vi "Experimentos de eletricidade.vi"() -> ()   [LabVIEW 2014]
panel:
  in  "Opções de aula":u16(ring) items=["Divisor de tensão.vi"]
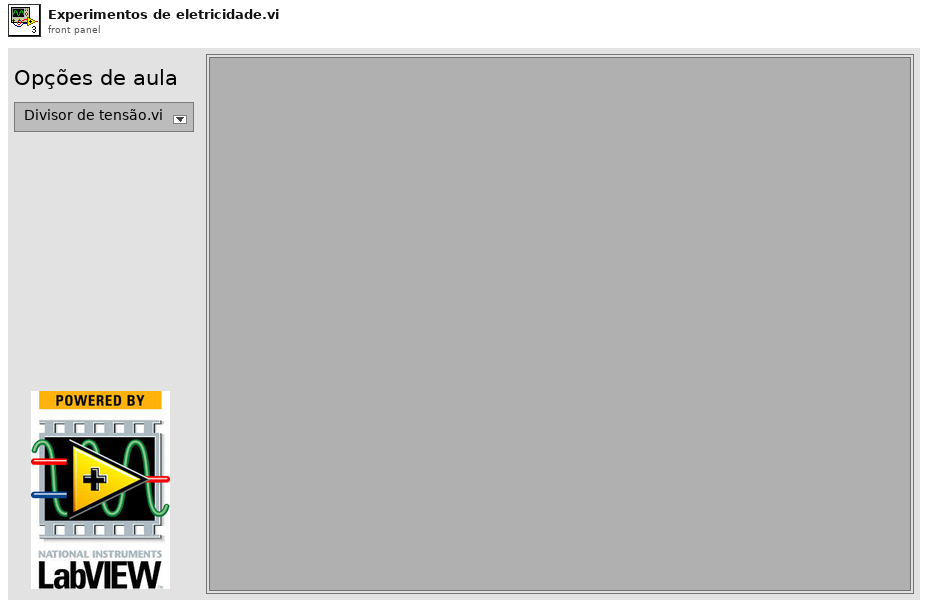
[diagram p1: front panel]
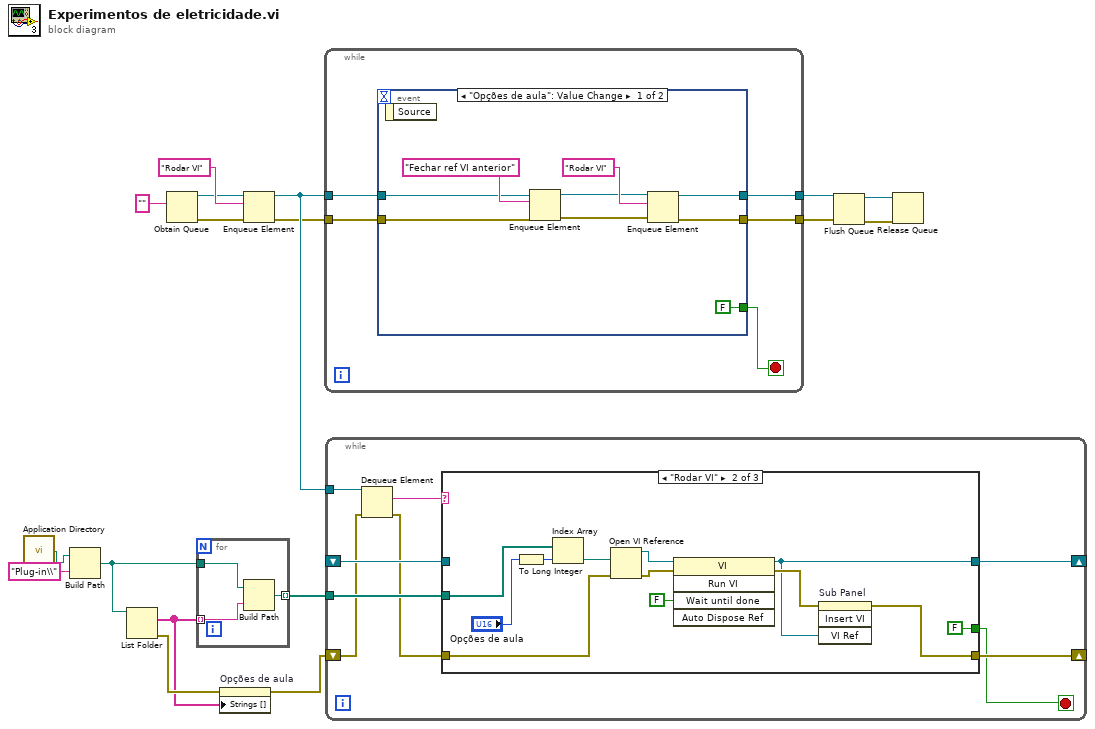
[diagram p0: block diagram]
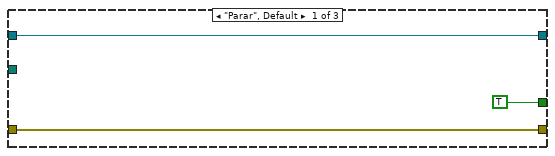
[diagram p2: hidden frame]
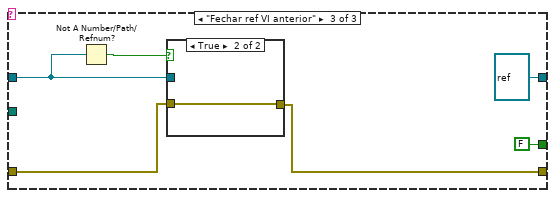
[diagram p3: hidden frame]
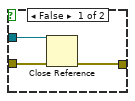
[diagram p4: hidden frame]
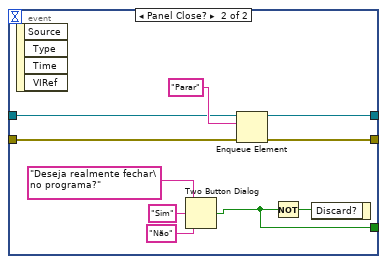
[diagram p5: hidden frame]
diagram:
  n1 = call <vilib>:"Application Directory.vi"() -> ("Application Directory"=w17:path)
  n2 = Build Path(base path=w17, name or relative path="Plug-in\\") -> (appended path=w15:path)
  n3 = List Folder(path=w15) -> (filenames=w13:string[], error out=w14:errorcluster)  [unwired: 3 in, 2 out]
  n4 = Obtain Queue(element data type="" ("name (unnamed)")) -> (queue out=w3:refnum<queue>, error out=w4:errorcluster)  [unwired: 4 in, 1 out]
  n5 = for {
    tunnel: w15 -> [w20]
    tunnel: w13 -> [w19] mode=indexing
    tunnel: [w18] -> w8 mode=indexing
    n6 = Build Path(base path=w20, name or relative path=w19) -> (appended path=w18:path)
  }
  n7 = property on="Opções de aula" class="Ring (strict)"(error in=w14, "Strings []"=w13) -> (error out=w7:errorcluster)  [unwired: 1 in, 1 out]
  n8 = Enqueue Element(queue=w3, element="Rodar VI", error in (no error)=w4) -> (queue out=w2:refnum<queue>, error out=w1:errorcluster)  [unwired: 1 in, 1 out]
  n9 = while {
    tunnel: w2 -> [w24]
    tunnel: w1 -> [w25]
    tunnel: [w23] -> w12
    tunnel: [w22] -> w11
    stop <- w21 stop-if-true
    n10 = event shown="[0] \"Opções de aula\": Value Change" {
      selector: _ -> [_ _]
      dyn-events: _ -> [_ _]
      timeout: _ -> [_ _]
      tunnel: w25 -> [w27 w35]
      tunnel: w24 -> [w28 w36]
      tunnel: [w34 w38] -> w23
      tunnel: [w33 w37] -> w22
      tunnel: [FALSE ("stop") w40] -> w21
      event "Opções de aula": Value Change {
        n11 = event-data() -> ()  [unwired: 1 in, 1 out]
        n12 = Enqueue Element(queue=w28, element="Fechar ref VI anterior", error in (no error)=w27) -> (queue out=w30:refnum<queue>, error out=w29:errorcluster)  [unwired: 1 in, 1 out]
        n13 = Enqueue Element(queue=w30, element="Rodar VI", error in (no error)=w29) -> (queue out=w34:refnum<queue>, error out=w33:errorcluster)  [unwired: 1 in, 1 out]
      }
      event Panel Close? {
        n14 = event-data() -> ()  [unwired: 1 in, 4 out]
        n15 = Two Button Dialog(message="Deseja realmente fechar\no programa?", 1:"Não" ("F button name (\"Cancel\")"), 2:"Sim" ("T button name (\"OK\")")) -> (T button?=w40:bool)
        n16 = Enqueue Element(queue=w36, element="Parar", error in (no error)=w35) -> (queue out=w38:refnum<queue>, error out=w37:errorcluster)  [unwired: 1 in, 1 out]
        n17 = Not(x=w40) -> (.not. x?=w41:bool)
        n18 = event-data("Discard?"=w41) -> ()  [unwired: 1 in, 1 out]
      }
    }
  }
  n19 = while {
    tunnel: w2 -> [w53]
    tunnel: w8 -> [w51]
    shift-right: [w50] -> _
    shift-left: _ -> [w49]
    shift-right: [w46] -> _
    shift-left: w7 -> [w48]
    stop <- w45 stop-if-true
    n20 = Dequeue Element(queue=w53, error in (no error)=w48) -> (element=w52:string, error out=w47:errorcluster)  [unwired: 1 in, 2 out]
    n21 = case shown="\"Rodar VI\"" w52 {
      tunnel: w51 -> [_ w63 _]
      tunnel: [w56 w61 refnum<vi> refnum ("vi reference")] -> w50
      tunnel: w47 -> [w55 w60 w74]
      tunnel: w49 -> [w56 _ w72]
      tunnel: [w55 w58 w70] -> w46
      tunnel: [TRUE FALSE FALSE] -> w45
      frame "Parar", Default {
      }
      frame "Rodar VI" {
        n22 = To Long Integer(number="Opções de aula") -> (32bit integer=w57:i32)
        n23 = Index Array(array=w63, index=w57) -> (element=w62:path)
        n24 = Open VI Reference(vi path=w62, error in (no error)=w60) -> (vi reference=w65:refnum<vi>, error out=w66:errorcluster)  [unwired: 4 in]
        n25 = invoke class="VI" method="Run VI"(reference=w65, error in=w66, "Wait until done"=FALSE ("Wait Until Done")) -> (reference out=w61:refnum<vi>, error out=w68:errorcluster)  [unwired: 2 in, 3 out]
        n26 = invoke on="Sub Panel" class="SubPanel" method="Insert VI"(error in=w68, "VI Ref"=w61) -> (error out=w58:errorcluster)  [unwired: 2 in, 3 out]
      }
      frame "Fechar ref VI anterior" {
        n27 = Not A Number/Path/Refnum?(number/path/refnum=w72) -> (NaN/Path/Refnum?=w73:bool)
        n28 = case shown="True" w73 {
          tunnel: w74 -> [w77 w78]
          tunnel: [w76 w78] -> w70
          tunnel: w72 -> [w75 _]
          frame False {
            n29 = Close Reference(reference=w75, error in (no error)=w77) -> (error out=w76:errorcluster)
          }
          frame True {
          }
        }
      }
    }
  }
  n30 = Flush Queue(queue=w12, error in (no error)=w11) -> (queue out=w10:refnum<queue>, error out=w9:errorcluster)  [unwired: 1 out]
  n31 = Release Queue(queue=w10, error in (no error)=w9) -> ()  [unwired: 1 in, 3 out]
